vi "Request Sequence Status.vi"(8 "error in (no error)":errorcluster, 11 "Sequencing Control in":refnum<class "Sequencing Control.lvclass">) -> (0 "error out":errorcluster, 3 "Sequencing Control out":refnum<class "Sequencing Control.lvclass">)   [LabVIEW 2020, in "VolatusSeqGUI.lvlib" / "Sequencing Control.lvclass"]
uses:
  Sequencing Control.lvclass
  VolatusSeq/Sequencing Status JSON.ctl
  VolatusSeq/Sequence Status JSON.ctl
  Sequencing Control.lvclass/Sequencing Control.ctl
  <vilib>/httpClient/LabVIEWHTTPClient.lvlib
  VolatusSeq/VolatusSeq.lvlib
  <vilib>/Utility/miscctls.llb/LVMapReplaceAction.ctl
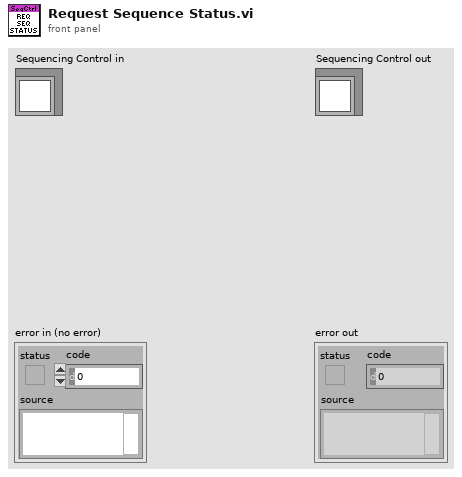
[diagram p1: front panel]
types:
  T1 = typedef "VolatusSeq.lvlib/Sequencing Status JSON.ctl" = cluster{"sequences":T2[]}
  T2 = typedef "VolatusSeq.lvlib/Sequence Status JSON.ctl" = cluster{"name":string, "state":string, "running":bool, "abort":bool, "time":cluster{"seq":i64, "state":i64, "wall":i64}, "loaded":bool, "started":i64, "crc":u32, "color_bg":string, "error":errorcluster}
  T3 = typedef "LVMapReplaceAction.ctl" = enum32{"Modify Entry only if found", "Add or Modify Entry", "Delete Entry"}
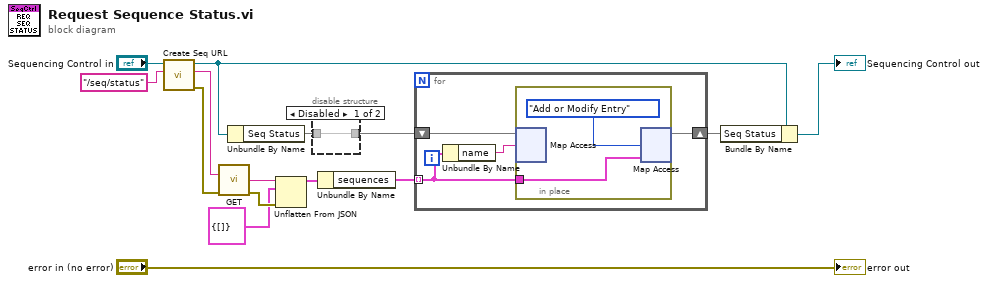
[diagram p0: block diagram]
diagram:
  n1 = call "Create Seq URL.vi"("Path"="/seq/status", "Sequencing Control in"="Sequencing Control in") -> ("error out"=w11:errorcluster, "Request URL"=w12:string, "Sequencing Control out"=w7:refnum<class "Sequencing Control.lvclass">)  [unwired: 7 in]
  n2 = call <vilib>:"GET.vi"("url"=w12, "error in (no error)"=w11) -> ("body"=w10:string, "error out"=w9:errorcluster)  [unwired: 10 in, 2 out]
  n3 = Unbundle By Name(w7) -> ("Seq Status"=w6:map{string, T2})
  n4 = Unflatten From JSON(JSON string=w10, type and defaults=T1 {"sequences"=[]} ("Sequencing Status JSON"), error in (no error)=w9) -> (value=w5:T1)  [unwired: 4 in, 1 out]
  n5 = disable-structure shown="Disabled" {
    disable-tunnel: [w16 _] -> w3
    disable-tunnel: w6 -> [w16 _]
    frame Disabled {
    }
    frame Enabled {
    }
  }
  n6 = Unbundle By Name(w5) -> ("sequences"=w4:T2[])
  n7 = for {
    tunnel: w4 -> [w18] mode=indexing
    shift-right: [w17] -> w1
    shift-left: w3 -> [w20]
    n8 = Unbundle By Name(w18) -> ("name"=w19:string)
    n9 = in-place {
      in-place-border: w18 -> [w21]
      n10 = in-place-map #1(w20, w19) -> ()  [unwired: 1 in, 2 out]
      n11 = in-place-map #1(w21, LVMapReplaceAction."Add or Modify Entry" ("action")) -> (w17:map{string, T2})  [unwired: 2 out]
    }
  }
  n12 = Bundle By Name(cluster=w7, "Seq Status"=w1) -> (→"Sequencing Control out":refnum<class "Sequencing Control.lvclass">)
  "error out" <- "error in (no error)"
